vi "GetBufferImageDimensions.vi"(8 "error in (no error)":errorcluster, 11 "Data Value Reference in":refnum<data-value>) -> (0 "error out":errorcluster, 3 "Dims":T1)   [LabVIEW 2020, in "Buffer.lvclass"]
uses:
  Buffer.lvclass
  Image Size.ctl
  Buffer.lvclass/Buffer.ctl
  bin/gindustrialcam_32-1.dll
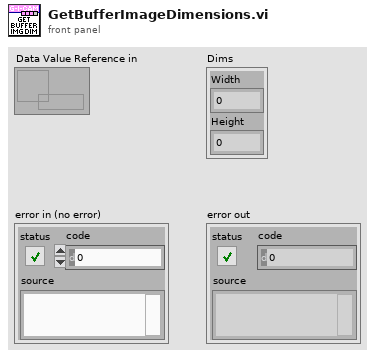
[diagram p1: front panel]
types:
  T1 = typedef "Buffer.lvclass/Image Size.ctl" = cluster{"Width":u16, "Height":u16}
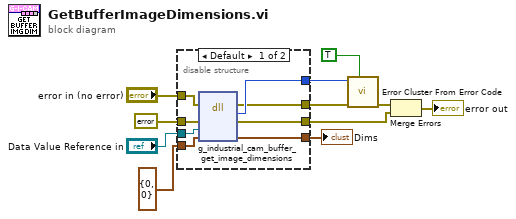
[diagram p0: block diagram]
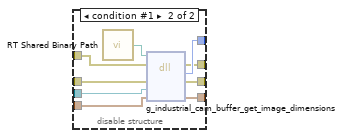
[diagram p2: hidden frame]
diagram:
  n1 = disable-structure shown="Default" {
    disable-tunnel: "Data Value Reference in" -> [w19 w28]
    disable-tunnel: [w18 w27] -> w10
    disable-tunnel: T1 {"Width"=0, "Height"=0} ("Image Size") -> [w17 w26]
    disable-tunnel: "error in (no error)" -> [w16 w25]
    disable-tunnel: errorcluster {"status"=FALSE, "code"=0, "source"=""} ("error constant") -> [w15 w24]
    disable-tunnel: [w14 w23] -> w4
    disable-tunnel: [w13 w22] -> w2
    disable-tunnel: [w12 w21] -> w1
    frame condition #0 (active) {
      n2 = dll-call lib="C:/serenial/lib/g-industrial-camera/LabVIEW/g_industrial_cam/bin/gindustrialcam_*-1.*" fn="g_industrial_cam_buffer_get_image_dimensions"(error in=w16, "err"=w15, "edvr"=w19, "dims"=w17) -> (error out=w12:errorcluster, "Mg_Error"=w13:i32, "err"=w14:errorcluster, "dims"=w18:T1)  [unwired: 3 in, 1 out]
    }
    frame condition #1 {
      n3 = call "RT Shared Binary Path.vi"() -> ("Path"=w20:path)
      n4 = dll-call lib="C:/serenial/lib/g-industrial-camera/LabVIEW/g_industrial_cam/bin/gindustrialcam_*-1.*" fn="g_industrial_cam_buffer_get_image_dimensions"(path in=w20, error in=w25, "err"=w24, "edvr"=w28, "dims"=w26) -> (error out=w21:errorcluster, "Mg_Error"=w22:i32, "err"=w23:errorcluster, "dims"=w27:T1)  [unwired: 2 in, 1 out]
    }
  }
  "Dims" <- w10
  n5 = call <vilib>:"Error Cluster From Error Code.vi"("show call chain? (False)"=TRUE, "error in (no error)"=w1, "error code (0)"=w2) -> ("error out"=w3:errorcluster)  [unwired: 6 in]
  n6 = Merge Errors(w3, w4) -> (→"error out":errorcluster)
